vi "Teststep1.vi"() -> ()   [LabVIEW 2019]
uses:
  <vilib>/Utility/error.llb/DialogType.ctl
  <vilib>/DAQmx/read.llb/DAQmx Read (Analog 1D Wfm NChan NSamp).vi
  <vilib>/DAQmx/write.llb/DAQmx Write (Analog 1D Wfm NChan NSamp).vi
  <vilib>/DAQmx/create/channels.llb/DAQmx Create Channel (AI-Acceleration-Accelerometer).vi
  <vilib>/DAQmx/create/channels.llb/DAQmx Create Channel (AI-Force-IEPE Sensor).vi
  <vilib>/DAQmx/create/channels.llb/DAQmx Create Channel (AI-Sound Pressure-Microphone).vi
  <vilib>/DAQmx/configure/timing.llb/DAQmx Timing (Sample Clock).vi
  <vilib>/DAQmx/configure/task.llb/DAQmx Configure Logging (TDMS).vi
  <vilib>/DAQmx/configure/trigger.llb/DAQmx Start Trigger (Digital Edge).vi
  <vilib>/DAQmx/configure/trigger.llb/DAQmx Start Trigger (Time).vi
  <vilib>/DAQmx/configure/trigger.llb/DAQmx Start Trigger (Analog Edge).vi
  <vilib>/DAQmx/create/channels.llb/DAQmx Create Channel (AO-Voltage-Basic).vi
  <vilib>/DAQmx/miscellaneous.llb/DAQmx Fill In Error Info.vi
  <resource>/objmgr/daqmx.rc
panel:
  out "Array":dbl[](array[numeric])
  out "Numeric":dbl
  in  "Stop 2":bool
  in  "Sample Rate 2":dbl=1000.0
  in  "Sample Clock Source 2":tag="OnboardClock"
  in  "Max Voltage":dbl=5.0
  in  "Min Voltage":dbl=-5.0
  in  "Physical Channel(s)":tag="Dev1/ao0"
  in  "Trigger Type 2":T1(tab)
  in  "Digital Start Trigger Edge 2":i32(ring)=10280 caption="Edge" items=["Rising"=10280, "Falling"=10171]
  in  "Digital Start Trigger Source 2":tag="/Dev1/PFI0" caption="Source"
  in  "Digital Pause Trigger Pause When 2":i32(ring)=10192 caption="Pause When" items=["High"=10192, "Low"=10214]
  in  "Digital Pause Trigger Source 2":tag="/Dev1/PFI0" caption="Source"
  in  "Analog Start Trigger Level 2":dbl caption="Level" format="%0.2f"
  in  "Analog Start Trigger Hysteresis 2":dbl caption="Hysteresis" format="%.2f"
  in  "Analog Start Trigger Slope 2":i32(ring)=10280 caption="Slope" items=["Rising"=10280, "Falling"=10171]
  in  "Analog Start Trigger Source 2":string="APFI0" caption="Source"
  in  "Analog Pause Trigger Source 2":string="APFI0" caption="Source"
  in  "Analog Pause Trigger Pause When 2":i32(ring)=10093 caption="Pause When" items=["Above Level"=10093, "Below Level"=10107]
  in  "Analog Pause Trigger Level 2":dbl caption="Level" format="%.2f"
  in  "When 2":timestamp
  in  "Select Time\nManually 2":bool
  out "Actual Sample Rate 2":dbl=1000.0 format="%0.2f"
  in  "Trigger Type":T1(tab)
  in  "Digital Start Trigger Edge":i32(ring)=10280 caption="Edge" items=["Rising"=10280, "Falling"=10171]
  in  "Digital Start Trigger Source":tag="/Dev1/PFI0" caption="Source"
  in  "Digital Pause Trigger Pause When":i32(ring)=10192 caption="Pause When" items=["High"=10192, "Low"=10214]
  in  "Digital Pause Trigger Source":tag="/Dev1/PFI0" caption="Source"
  in  "Analog Start Trigger Level":dbl caption="Level" format="%0.2f"
  in  "Analog Start Trigger Hysteresis":dbl caption="Hysteresis" format="%.2f"
  in  "Analog Start Trigger Slope":i32(ring)=10280 caption="Slope" items=["Rising"=10280, "Falling"=10171]
  in  "Analog Start Trigger Source":string="APFI0" caption="Source"
  in  "Analog Pause Trigger Source":string="APFI0" caption="Source"
  in  "Analog Pause Trigger Pause When":i32(ring)=10093 caption="Pause When" items=["Above Level"=10093, "Below Level"=10107]
  in  "Analog Pause Trigger Level":dbl caption="Level" format="%.2f"
  in  "When":timestamp
  in  "Select Time\nManually":bool
  in  "IEPE Excitation Source":i32(ring)=10200 items=["Internal"=10200, "External"=10167, "None"=10230]
  in  "IEPE Current Value (A)":dbl=0.004
  in  "Terminal Configuration":i32(ring)=-1 items=["default"=-1, "RSE"=10083, "NRSE"=10078, "Differential"=10106, "Pseudodifferential"=12529]
  in  "Physical Channel":tag="Dev1/ai0"
  in  "Task Type":T2(tab)
  in  "Min Acceleration":dbl=-100.0
  in  "Max Acceleration":dbl=100.0
  in  "Sensitivity":dbl=50.0
  in  "Acceleration Units":i32(ring)=10186 items=["g"=10186, "m/s^2"=12470, "in/s^2"=12471, "From Custom Scale"=10065]
  in  "Sensitivity Units":i32(ring)=12509 items=["mVolts/g"=12509, "Volts/g"=12510]
  in  "Max Sound Pressure Level (dB)":dbl=120.0
  in  "Sound Pressure Units":i32(ring)=10081 items=["Pascals"=10081, "From Custom Scale"=10065]
  in  "Microphone Sensitivity":dbl=10.0
  in  "Sensitivity 2":dbl=50.0
  in  "Min Force":dbl=-100.0
  in  "Max Force":dbl=100.0
  in  "Sensitivity Units  2":i32(ring)=15891 items=["mVolts/N"=15891, "mVolts/lb"=15892]
  in  "Force Units":i32(ring)=15875 items=["Newtons"=15875, "Pounds"=15876, "From Custom Scale"=10065]
  in  "TDMS File Path":path
  in  "Sample Rate":dbl=1000.0
  in  "Sample Clock Source":tag="OnboardClock"
  out "Actual Sample Rate":dbl=1000.0000111176631 format="%0.2f"
  in  "Logging Mode":i32(ring)=10231 items=["Off"=10231, "Log and Read"=15842]
  in  "Samples per Loop":i32=100
  in  "Stop":bool
  out "Waveform Graph":waveform(dbl)[](graph)
  # "To enable triggers, select a tab above, and configure the settings.\n\nNot all hardware supports all trigger types. Refer to your device documentation for more information."
  # "This trigger type is not supported in output tasks. \n\nRefer to your device documentation for more information on which triggers are supported."
  # "This trigger type is not supported in output tasks. \n\nRefer to your device documentation for more information on which triggers are supported."
  # "If time is not manually set, task will begin after 10 seconds"
  # "To enable triggers, select a tab above, and configure the settings.\n\nNot all hardware supports all trigger types. Refer to your device documentation for more information."
  # "This trigger type is not supported in continuous sample timing. \n\nRefer to your device documentation for more information on which triggers are supported."
  # "This trigger type is not supported in continuous sample timing. \n\nRefer to your device documentation for more information on which triggers are supported."
  # "If time is not manually set, task will begin after 10 seconds"
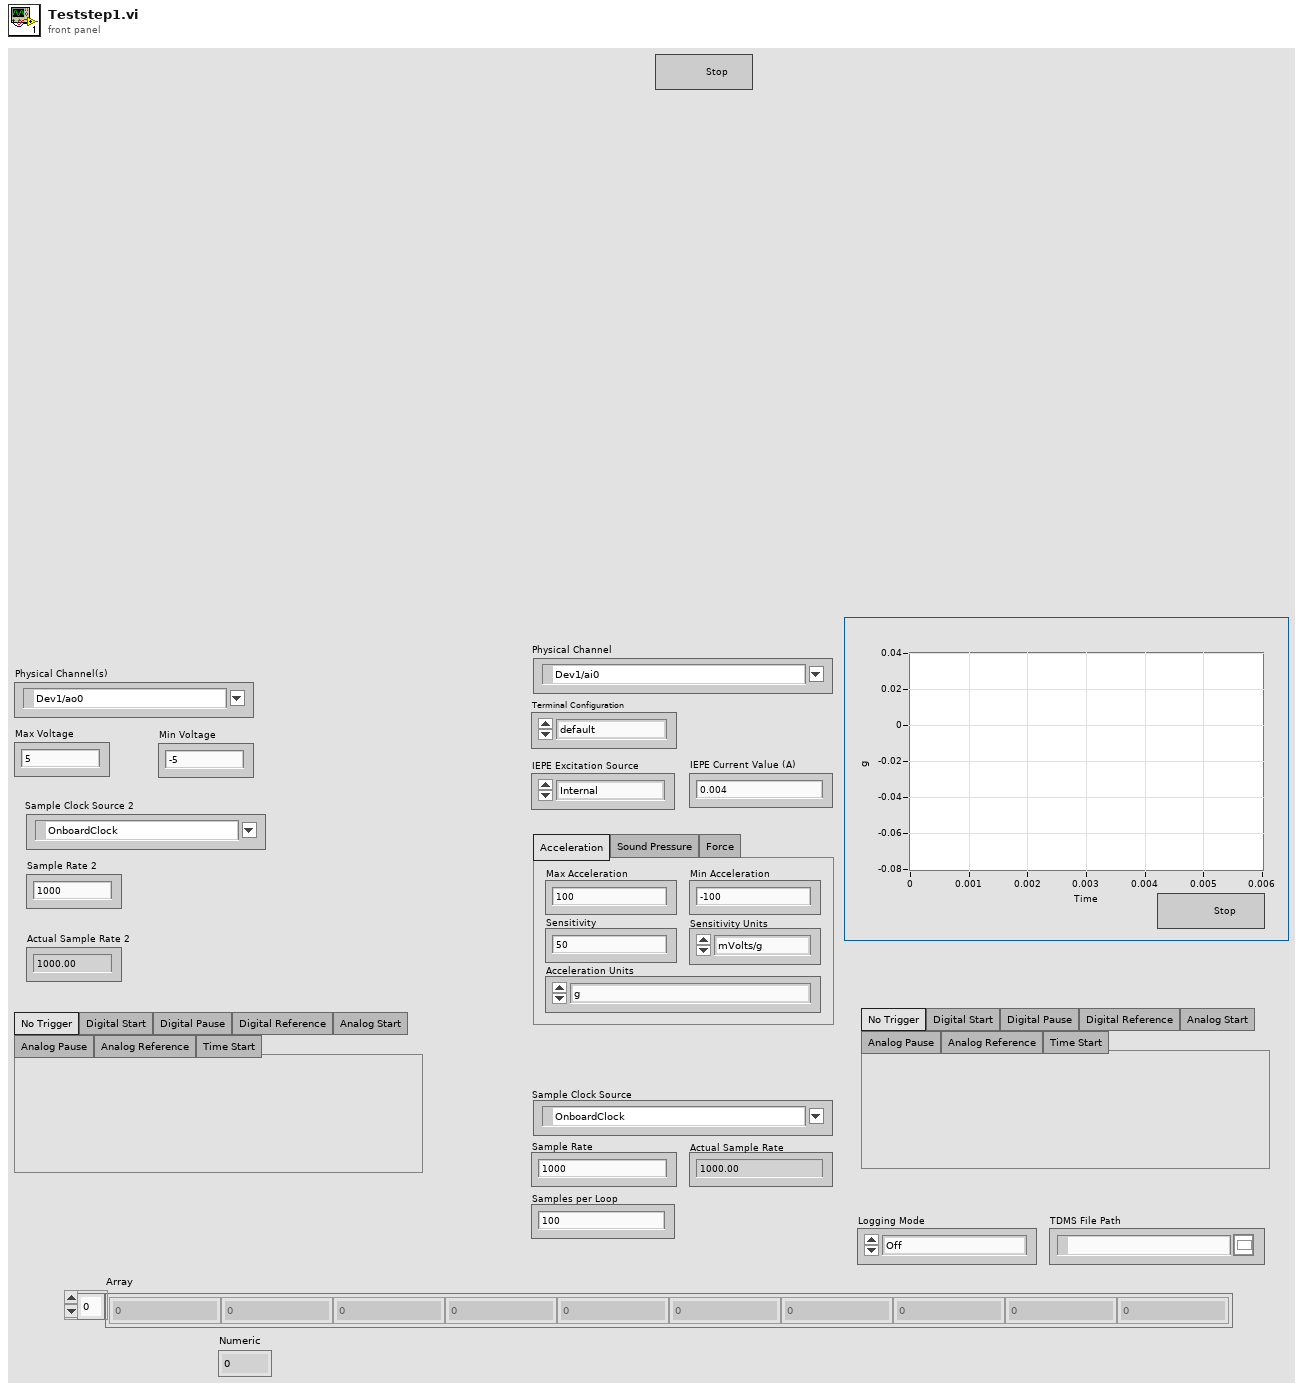
[diagram p1: front panel]
types:
  T1 = enum32{"No Trigger", "Digital Start", "Digital Pause", "Digital Reference", "Analog Start", "Analog Pause", "Analog Reference", "Time Start"}
  T2 = enum32{"Acceleration", "Sound Pressure", "Force"}
  T3 = typedef "DialogType.ctl" = u16
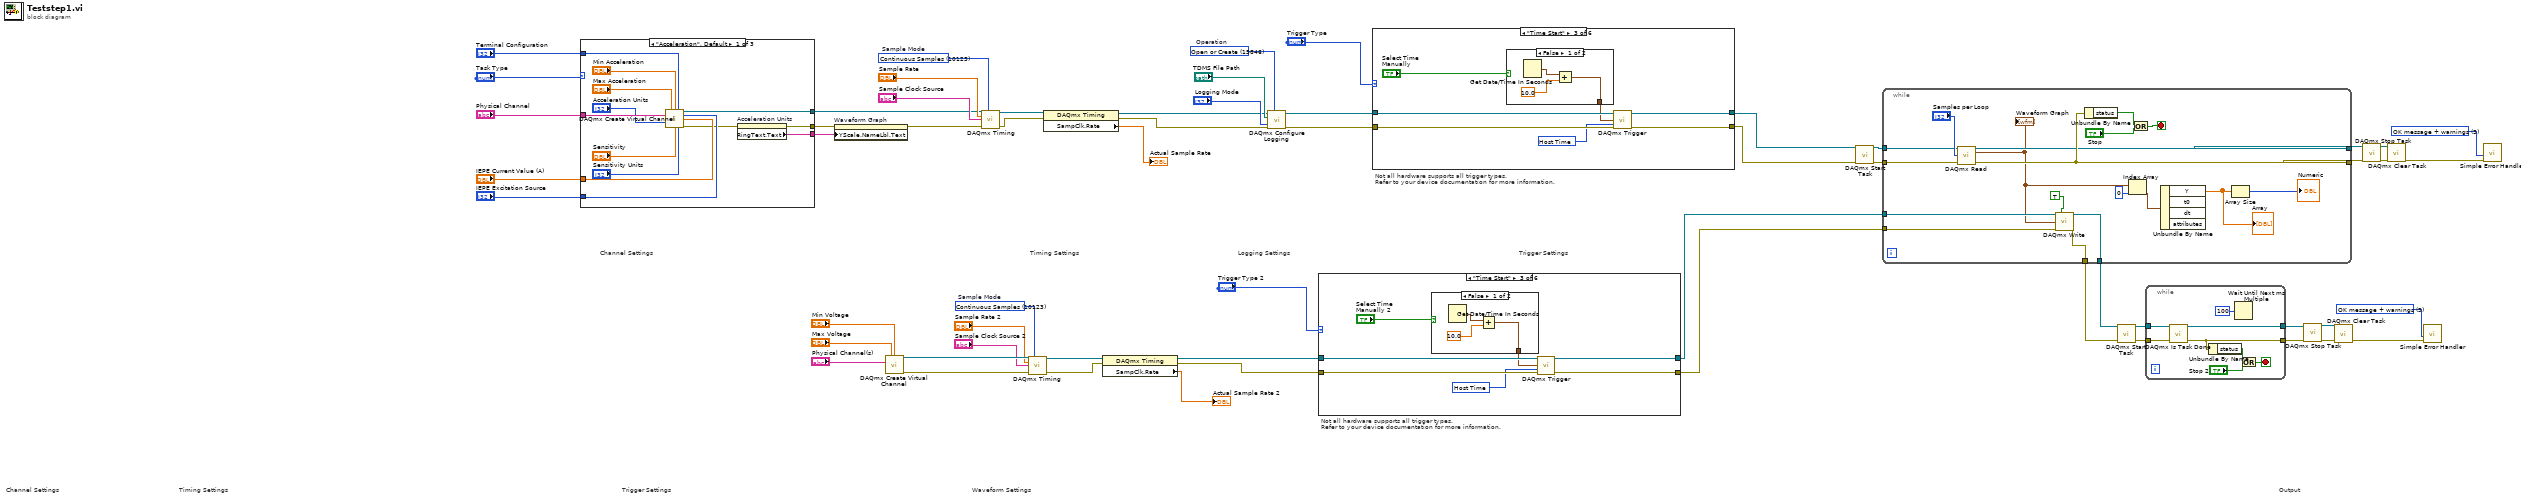
[diagram p0: block diagram]
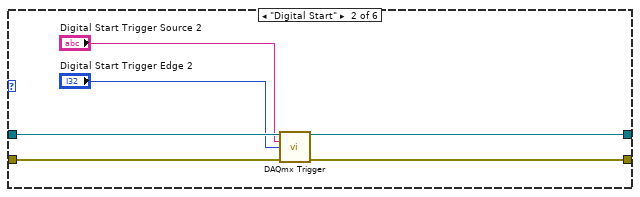
[diagram p3: hidden frame]
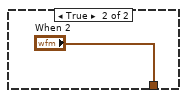
[diagram p4: hidden frame]
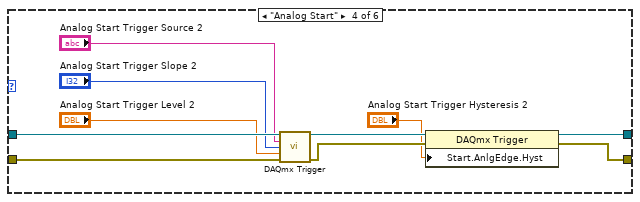
[diagram p5: hidden frame]
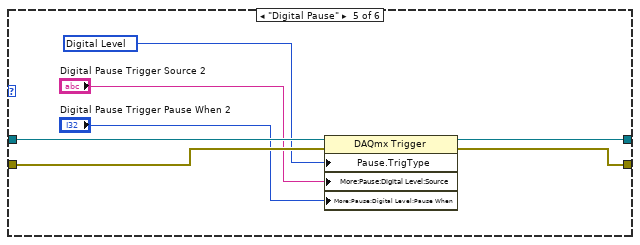
[diagram p6: hidden frame]
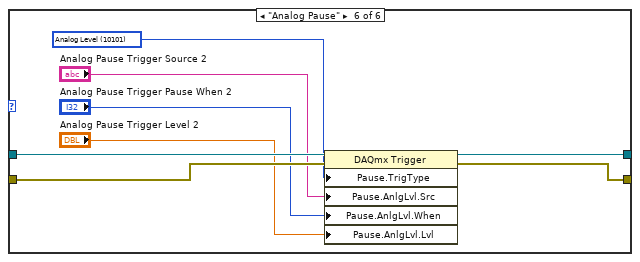
[diagram p7: hidden frame]
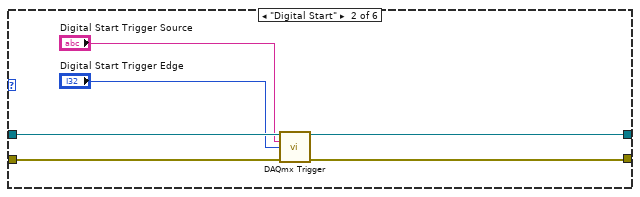
[diagram p9: hidden frame]
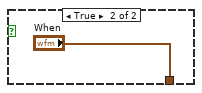
[diagram p10: hidden frame]
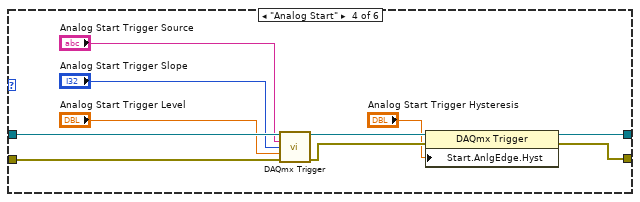
[diagram p11: hidden frame]
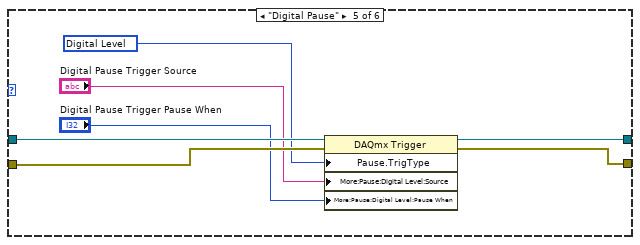
[diagram p12: hidden frame]
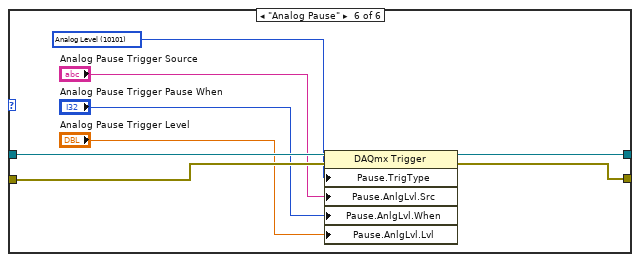
[diagram p13: hidden frame]
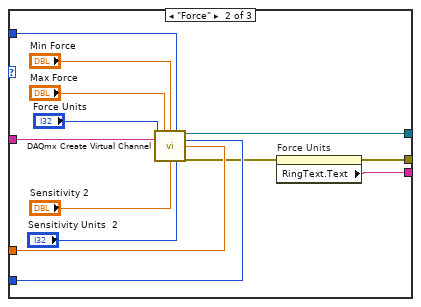
[diagram p14: hidden frame]
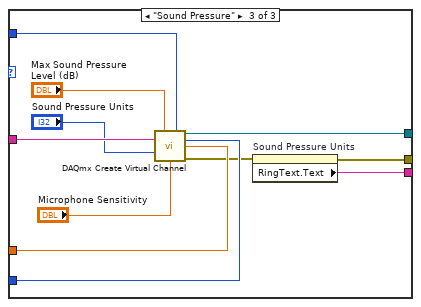
[diagram p15: hidden frame]
diagram:
  w3 = T3 3 items=["no dialog", "OK message", "continue or stop message", "OK message + warnings", "continue/stop + warnings"] ("type of dialog (OK msg:1)")
  w9 = T3 3 items=["no dialog", "OK message", "continue or stop message", "OK message + warnings", "continue/stop + warnings"] ("type of dialog (OK msg:1)")
  w32 = 10123 items=["Finite Samples"=10178, "Continuous Samples"=10123, "Hardware Timed Single Point"=12522]  # Sample Mode
  w58 = 15846 items=["Open"=10437, "Open or Create"=15846, "Create or Replace"=15847, "Create"=15848]  # Operation
  w59 = 10123 items=["Finite Samples"=10178, "Continuous Samples"=10123, "Hardware Timed Single Point"=12522]  # Sample Mode
  # "Not all hardware supports all trigger types.\nRefer to your device documentation for more information."
  # "Timing Settings"
  # "Channel Settings"
  # "Trigger Settings"
  # "Output"
  # "Waveform Settings"
  # "Trigger Settings"
  # "Not all hardware supports all trigger types.\nRefer to your device documentation for more information."
  # "Timing Settings"
  # "Channel Settings"
  # "Logging Settings"
  n1 = case shown="\"Acceleration\", Default" "Task Type" {
    tunnel: [w62 w75 w89] -> w44
    tunnel: [w72 w85 w96] -> w45
    tunnel: "Physical Channel" -> [w71 w84 w95]
    tunnel: "IEPE Excitation Source" -> [w70 w83 w91]
    tunnel: "IEPE Current Value (A)" -> [w69 w82 w92]
    tunnel: "Terminal Configuration" -> [w68 w81 w94]
    tunnel: [w60 w74 w88] -> w43
    frame "Acceleration", Default {
      n2 = call-poly <vilib>:"DAQmx Create Virtual Channel.vi"("maximum value"="Max Acceleration", "minimum value"="Min Acceleration", "input terminal configuration"=w68, "physical channels"=w71, "current excitation source"=w70, "current excitation value"=w69, "units"="Acceleration Units", "sensitivity"="Sensitivity", "sensitivity units"="Sensitivity Units") -> ("task out"=w72:refnum<k21>, "error out"=w61:errorcluster)  [unwired: 5 in]
      n3 = property on="Acceleration Units" class="Ring (strict)"(error in=w61) -> (error out=w62:errorcluster, "RingText.Text"=w60:string)  [unwired: 1 in, 1 out]
    }
    frame "Force" {
      n4 = call-poly <vilib>:"DAQmx Create Virtual Channel.vi"("maximum value"="Max Force", "minimum value"="Min Force", "input terminal configuration"=w81, "physical channels"=w84, "current excitation source"=w83, "current excitation value"=w82, "units"="Force Units", "sensitivity"="Sensitivity 2", "sensitivity units"="Sensitivity Units  2") -> ("task out"=w85:refnum<k21>, "error out"=w73:errorcluster)  [unwired: 5 in]
      n5 = property on="Force Units" class="Ring (strict)"(error in=w73) -> (error out=w75:errorcluster, "RingText.Text"=w74:string)  [unwired: 1 in, 1 out]
    }
    frame "Sound Pressure" {
      n6 = call-poly <vilib>:"DAQmx Create Virtual Channel.vi"("maximum sound pressure level"="Max Sound Pressure Level (dB)", "input terminal configuration"=w94, "physical channels"=w95, "current excitation source"=w91, "current excitation value"=w92, "units"="Sound Pressure Units", "microphone sensitivity"="Microphone Sensitivity") -> ("task out"=w96:refnum<k21>, "error out"=w87:errorcluster)  [unwired: 7 in]
      n7 = property on="Sound Pressure Units" class="Ring (strict)"(error in=w87) -> (error out=w89:errorcluster, "RingText.Text"=w88:string)  [unwired: 1 in, 1 out]
    }
  }
  n8 = property on="Waveform Graph" class="WFGraph (strict)"(error in=w44, "YScale.NameLbl.Text"=w43) -> (error out=w42:errorcluster)  [unwired: 1 in, 1 out]
  n9 = call-poly <vilib>:"DAQmx Create Virtual Channel.vi"("maximum value"="Max Voltage", "minimum value"="Min Voltage", "physical channels"="Physical Channel(s)") -> ("task out"=w30:refnum<k21>, "error out"=w31:errorcluster)  [unwired: 11 in]
  n10 = call-poly <vilib>:"DAQmx Timing.vi"("task/channels in"=w45, "sample mode"=w59, "rate"="Sample Rate", "source"="Sample Clock Source", "error in"=w42) -> ("task out"=w37:refnum<k21>, "error out"=w36:errorcluster)  [unwired: 9 in]
  n11 = call-poly <vilib>:"DAQmx Timing.vi"("task/channels in"=w30, "sample mode"=w32, "rate"="Sample Rate 2", "source"="Sample Clock Source 2", "error in"=w31) -> ("task out"=w24:refnum<k21>, "error out"=w23:errorcluster)  [unwired: 9 in]
  n12 = property class="DAQmx Timing"(reference=w37, error in=w36) -> (reference out=w35:refnum<k21>, error out=w34:errorcluster, "SampClk.Rate"=→"Actual Sample Rate":dbl)
  n13 = property class="DAQmx Timing"(reference=w24, error in=w23) -> (reference out=w22:refnum<k21>, error out=w21:errorcluster, "SampClk.Rate"=→"Actual Sample Rate 2":dbl)
  n14 = call-poly <vilib>:"DAQmx Configure Logging.vi"("task/channels in"=w35, "operation"=w58, "file path"="TDMS File Path", "logging mode"="Logging Mode", "error in"=w34) -> ("task out"=w39:refnum<k21>, "error out"=w40:errorcluster)  [unwired: 9 in]
  n15 = case shown="\"Time Start\"" "Trigger Type 2" {
    tunnel: w22 -> [w98 w104 w111 w125 w132 w140]
    tunnel: w21 -> [w97 w103 w110 w124 w129 w137]
    tunnel: [w98 w102 w109 w122 w131 w139] -> w19
    tunnel: [w97 w101 w108 w121 w130 w138] -> w18
    frame "No Trigger", Default {
    }
    frame "Digital Start" {
      n16 = call-poly <vilib>:"DAQmx Trigger.vi"("task/channels in"=w104, "source"="Digital Start Trigger Source 2", "edge"="Digital Start Trigger Edge 2", "error in"=w103) -> ("task out"=w102:refnum<k21>, "error out"=w101:errorcluster)  [unwired: 10 in]
    }
    frame "Time Start" {
      w107 = 16126 items=["Host Time"=16126, "I/O Device Time"=16127] ("timescale")
      n17 = case shown="False" "Select Time\nManually 2" {
        tunnel: [w113 "When 2"] -> w105
        frame False {
          n18 = Get Date/Time In Seconds() -> (seconds since 1Jan1904=w114:timestamp)
          n19 = Add(x=w114, y=10.0) -> (x+y=w113:timestamp)
        }
        frame True {
        }
      }
      n20 = call-poly <vilib>:"DAQmx Trigger.vi"("task/channels in"=w111, "when"=w105, "timescale"=w107, "error in"=w110) -> ("task out"=w109:refnum<k21>, "error out"=w108:errorcluster)  [unwired: 10 in]
    }
    frame "Analog Start" {
      n21 = call-poly <vilib>:"DAQmx Trigger.vi"("task/channels in"=w125, "source"="Analog Start Trigger Source 2", "slope"="Analog Start Trigger Slope 2", "level"="Analog Start Trigger Level 2", "error in"=w124) -> ("task out"=w120:refnum<k21>, "error out"=w119:errorcluster)  [unwired: 9 in]
      n22 = property class="DAQmx Trigger"(reference=w120, error in=w119, "Start.AnlgEdge.Hyst"="Analog Start Trigger Hysteresis 2") -> (reference out=w122:refnum<k21>, error out=w121:errorcluster)
    }
    frame "Digital Pause" {
      w128 = 10152 items=["Analog Level"=10101, "Analog Window"=10103, "Digital Level"=10152, "Digital Pattern"=10398, "None"=10230] ("Pause.TrigType")
      n23 = property class="DAQmx Trigger"(reference=w132, error in=w129, "Pause.TrigType"=w128, "More:Pause:Digital Level:Source"="Digital Pause Trigger Source 2", "More:Pause:Digital Level:Pause When"="Digital Pause Trigger Pause When 2") -> (reference out=w131:refnum<k21>, error out=w130:errorcluster)
    }
    frame "Analog Pause" {
      w136 = 10101 items=["Analog Level"=10101, "Analog Window"=10103, "Digital Level"=10152, "Digital Pattern"=10398, "None"=10230] ("Pause.TrigType")
      n24 = property class="DAQmx Trigger"(reference=w140, error in=w137, "Pause.TrigType"=w136, "Pause.AnlgLvl.Src"="Analog Pause Trigger Source 2", "Pause.AnlgLvl.When"="Analog Pause Trigger Pause When 2", "Pause.AnlgLvl.Lvl"="Analog Pause Trigger Level 2") -> (reference out=w139:refnum<k21>, error out=w138:errorcluster)
    }
  }
  n25 = case shown="\"Time Start\"" "Trigger Type" {
    tunnel: w39 -> [w142 w148 w155 w169 w176 w184]
    tunnel: w40 -> [w141 w147 w154 w168 w173 w181]
    tunnel: [w142 w146 w153 w166 w175 w183] -> w17
    tunnel: [w141 w145 w152 w165 w174 w182] -> w38
    frame "No Trigger", Default {
    }
    frame "Digital Start" {
      n26 = call-poly <vilib>:"DAQmx Trigger.vi"("task/channels in"=w148, "source"="Digital Start Trigger Source", "edge"="Digital Start Trigger Edge", "error in"=w147) -> ("task out"=w146:refnum<k21>, "error out"=w145:errorcluster)  [unwired: 10 in]
    }
    frame "Time Start" {
      w149 = 16126 items=["Host Time"=16126, "I/O Device Time"=16127] ("timescale")
      n27 = case shown="False" "Select Time\nManually" {
        tunnel: [w157 "When"] -> w150
        frame False {
          n28 = Get Date/Time In Seconds() -> (seconds since 1Jan1904=w158:timestamp)
          n29 = Add(x=w158, y=10.0) -> (x+y=w157:timestamp)
        }
        frame True {
        }
      }
      n30 = call-poly <vilib>:"DAQmx Trigger.vi"("task/channels in"=w155, "when"=w150, "timescale"=w149, "error in"=w154) -> ("task out"=w153:refnum<k21>, "error out"=w152:errorcluster)  [unwired: 10 in]
    }
    frame "Analog Start" {
      n31 = call-poly <vilib>:"DAQmx Trigger.vi"("task/channels in"=w169, "source"="Analog Start Trigger Source", "slope"="Analog Start Trigger Slope", "level"="Analog Start Trigger Level", "error in"=w168) -> ("task out"=w164:refnum<k21>, "error out"=w163:errorcluster)  [unwired: 9 in]
      n32 = property class="DAQmx Trigger"(reference=w164, error in=w163, "Start.AnlgEdge.Hyst"="Analog Start Trigger Hysteresis") -> (reference out=w166:refnum<k21>, error out=w165:errorcluster)
    }
    frame "Digital Pause" {
      w172 = 10152 items=["Analog Level"=10101, "Analog Window"=10103, "Digital Level"=10152, "Digital Pattern"=10398, "None"=10230] ("Pause.TrigType")
      n33 = property class="DAQmx Trigger"(reference=w176, error in=w173, "Pause.TrigType"=w172, "More:Pause:Digital Level:Source"="Digital Pause Trigger Source", "More:Pause:Digital Level:Pause When"="Digital Pause Trigger Pause When") -> (reference out=w175:refnum<k21>, error out=w174:errorcluster)
    }
    frame "Analog Pause" {
      w180 = 10101 items=["Analog Level"=10101, "Analog Window"=10103, "Digital Level"=10152, "Digital Pattern"=10398, "None"=10230] ("Pause.TrigType")
      n34 = property class="DAQmx Trigger"(reference=w184, error in=w181, "Pause.TrigType"=w180, "Pause.AnlgLvl.Src"="Analog Pause Trigger Source", "Pause.AnlgLvl.When"="Analog Pause Trigger Pause When", "Pause.AnlgLvl.Lvl"="Analog Pause Trigger Level") -> (reference out=w183:refnum<k21>, error out=w182:errorcluster)
    }
  }
  n35 = call <vilib>:"DAQmx Start Task.vi"("task/channels in"=w17, "error in"=w38) -> ("task out"=w57:refnum<k21>, "error out"=w56:errorcluster)  [unwired: 12 in]
  n36 = while {
    tunnel: w57 -> [w197]
    tunnel: w56 -> [w202]
    tunnel: [w195] -> w2
    tunnel: w19 -> [w194]
    tunnel: w18 -> [w196]
    tunnel: [w193] -> w8
    tunnel: [w192] -> w7
    tunnel: [w191] -> w1
    stop <- w201 stop-if-true
    n37 = call-poly <vilib>:"DAQmx Read.vi"("task/channels in"=w197, "number of samples per channel"="Samples per Loop", "error in"=w202) -> ("task out"=w191:refnum<k21>, "data"=w189:waveform(dbl)[], "error out"=w195:errorcluster)  [unwired: 10 in]
    "Waveform Graph" <- w189
    n38 = call-poly <vilib>:"DAQmx Write.vi"("task/channels in"=w194, "auto start"=TRUE, "data"=w189, "error in"=w196) -> ("task out"=w193:refnum<k21>, "error out"=w192:errorcluster)  [unwired: 9 in, 1 out]
    n39 = Unbundle By Name(w195) -> ("status"=w200:bool)
    n40 = Index Array(array=w189, index=0) -> (element=w187:waveform(dbl))
    n41 = Or(x=w200, y="Stop") -> (x .or. y?=w201:bool)
    n42 = Unbundle By Name(w187) -> ("Y"=w185:dbl[])  [unwired: 3 out]
    "Array" <- w185
    n43 = Array Size(array=w185) -> (size(s)=→"Numeric":i32)
  }
  n44 = call <vilib>:"DAQmx Start Task.vi"("task/channels in"=w8, "error in"=w7) -> ("task out"=w16:refnum<k21>, "error out"=w15:errorcluster)  [unwired: 12 in]
  n45 = while {
    tunnel: w16 -> [w210]
    tunnel: w15 -> [w209]
    tunnel: [w206] -> w10
    tunnel: [w207] -> w11
    stop <- w208 stop-if-true
    n46 = call <vilib>:"DAQmx Is Task Done.vi"("task/channels in"=w210, "error in"=w209) -> ("task out"=w207:refnum<k21>, "error out"=w206:errorcluster)  [unwired: 11 in, 1 out]
    n47 = Unbundle By Name(w206) -> ("status"=w205:bool)
    n48 = Wait Until Next ms Multiple(millisecond multiple=u32 100) -> ()  [unwired: 1 out]
    n49 = Or(x=w205, y="Stop 2") -> (x .or. y?=w208:bool)
  }
  n50 = call <vilib>:"DAQmx Stop Task.vi"("task/channels in"=w11, "error in"=w10) -> ("task out"=w13:refnum<k21>, "error out"=w12:errorcluster)  [unwired: 12 in]
  n51 = call <vilib>:"DAQmx Clear Task.vi"("task in"=w13, "error in"=w12) -> ("error out"=w14:errorcluster)  [unwired: 13 in]
  n52 = call <vilib>:"DAQmx Stop Task.vi"("task/channels in"=w1, "error in"=w2) -> ("task out"=w5:refnum<k21>, "error out"=w4:errorcluster)  [unwired: 12 in]
  n53 = call <vilib>:"DAQmx Clear Task.vi"("task in"=w5, "error in"=w4) -> ("error out"=w6:errorcluster)  [unwired: 13 in]
  n54 = call <vilib>:"Simple Error Handler.vi"("type of dialog (OK msg:1)"=w9, "error in (no error)"=w14) -> ()  [unwired: 3 in, 5 out]
  n55 = call <vilib>:"Simple Error Handler.vi"("type of dialog (OK msg:1)"=w3, "error in (no error)"=w6) -> ()  [unwired: 3 in, 5 out]
